vi "tcpExampleSelfContained.vi"() -> ()   [LabVIEW 2014]
uses:
  typedefs/clientStatus.ctl
  typedefs/clientConfiguration.ctl
panel:
  out "server status":T1
  out "receive server->client":string
  out "receive client->server":string
  in  "transmit client->server":string
  in  "transmit server->client":string
  in  "stop":bool
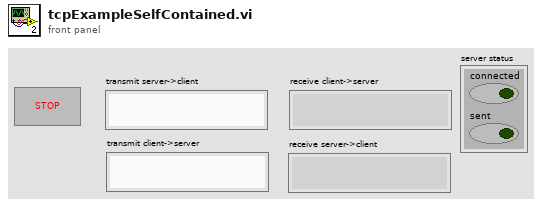
[diagram p1: front panel]
types:
  T1 = typedef "clientStatus.ctl" = cluster{"connected":bool, "sent":bool}
  T2 = typedef "clientConfiguration.ctl" = cluster{"client ID":string, "remote host":string, "local port":u16, "remote port":u16}
  T3 = typedef "QueueCluster.ctl" = cluster{"status":cluster{"queue":refnum<queue>, "error out":errorcluster}, "receive":cluster{"queue":refnum<queue>, "error out":errorcluster}, "transmit":cluster{"queue":refnum<queue>, "error out":errorcluster}, "shutdown":cluster{"queue":refnum<queue>, "error out":errorcluster}, "semaphore":T4}
  T4 = typedef "Semaphore RefNum" = refnum<k1>
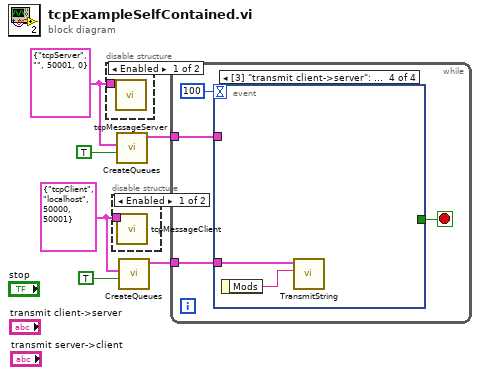
[diagram p0: block diagram]
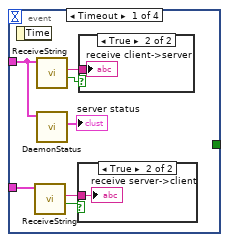
[diagram p4: hidden frame]
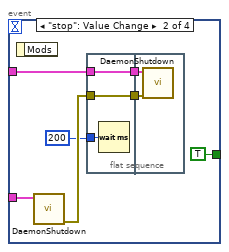
[diagram p7: hidden frame]
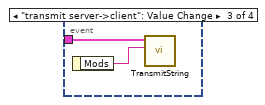
[diagram p8: hidden frame]
diagram:
  w6 = T2 {"client ID"="tcpClient", "remote host"="localhost", "local port"=50000, "remote port"=50001} ("client configuration")
  w5 = T2 {"client ID"="tcpServer", "remote host"="", "local port"=50001, "remote port"=0} ("client configuration")
  n1 = disable-structure shown="Enabled" {
    disable-tunnel: w5 -> [w7 _]
    frame Enabled {
      n2 = call "tcpMessageServer.vi"("server configuration"=w7) -> ()  [unwired: 10 in, 1 out]
    }
    frame Disabled {
    }
  }
  n3 = disable-structure shown="Enabled" {
    disable-tunnel: w6 -> [w8 _]
    frame Enabled {
      n4 = call "tcpMessageClient.vi"("client configuration"=w8) -> ()  [unwired: 10 in, 1 out]
    }
    frame Disabled {
    }
  }
  n5 = call "CreateQueues.vi"("create if not found? (T)"=TRUE, "client configuration"=w5) -> ("output cluster"=w2:T3)  [unwired: 9 in]
  n6 = call "CreateQueues.vi"("create if not found? (T)"=TRUE, "client configuration"=w6) -> ("output cluster"=w1:T3)  [unwired: 9 in]
  n7 = while {
    tunnel: w2 -> [w11]
    tunnel: w1 -> [w10]
    stop <- w12 stop-if-true
    n8 = event shown="[3] \"transmit client->server\": Key Up" {
      selector: _ -> [_ _ _ _]
      dyn-events: _ -> [_ _ _ _]
      timeout: 100 -> [_ _ _ _]
      tunnel: [_ TRUE _ _] -> w12
      tunnel: w11 -> [w16 w27 w35 _]
      tunnel: w10 -> [w19 w26 _ w36]
      event Timeout {
        n9 = event-data() -> ()  [unwired: 1 in, 1 out]
        n10 = call "ReceiveString.vi"("queue cluster"=w19) -> ("new value"=w14:bool, "received string"=w17:string)  [unwired: 7 in, 2 out]
        n11 = call "ReceiveString.vi"("queue cluster"=w16) -> ("new value"=w13:bool, "received string"=w18:string)  [unwired: 7 in, 2 out]
        n12 = call "DaemonStatus.vi"("queue cluster"=w16) -> ("status"=→"server status":T1)  [unwired: 8 in, 2 out]
        n13 = case shown="True" w14 {
          tunnel: w17 -> [_ w21]
          frame False {
          }
          frame True {
            "receive server->client" <- w21
          }
        }
        n14 = case shown="True" w13 {
          tunnel: w18 -> [_ w20]
          frame False {
          }
          frame True {
            "receive client->server" <- w20
          }
        }
      }
      event "stop": Value Change {
        n15 = event-data() -> ()  [unwired: 1 in, 1 out]
        n16 = call "DaemonShutdown.vi"("queue cluster"=w26) -> ("error out"=w23:errorcluster)  [unwired: 9 in, 1 out]
        n17 = flat-sequence {
          tunnel: w27 -> [w31]
          tunnel: [w31] -> w25
          tunnel: [w30] -> w24
          tunnel: w23 -> [w30]
          tunnel: 200 -> [w29]
          tunnel: w25 -> [w33]
          tunnel: w24 -> [w32]
          frame #0 {
            n18 = Wait (ms)(milliseconds to wait=w29) -> ()  [unwired: 1 out]
          }
          frame #1 {
            n19 = call "DaemonShutdown.vi"("error in (no error)"=w32, "queue cluster"=w33) -> ()  [unwired: 8 in, 2 out]
          }
        }
      }
      event "transmit server->client": Value Change {
        n20 = event-data() -> ("Mods"=w34:string)  [unwired: 1 in]
        n21 = call "TransmitString.vi"("string to transmit"=w34, "queue cluster"=w35) -> ()  [unwired: 8 in, 2 out]
      }
      event "transmit client->server": Value Change {
        n22 = event-data() -> ("Mods"=w37:string)  [unwired: 1 in]
        n23 = call "TransmitString.vi"("string to transmit"=w37, "queue cluster"=w36) -> ()  [unwired: 8 in, 2 out]
      }
    }
  }
